vi "Polynomial Roots (CDB).vi"(10 "option":u16(ring) items=["General"=0, "Advanced Refinement"=3], 11 "P(x)":cdb[](array[numeric]) format="%#.6g") -> (0 "error":i32, 3 "Roots":cdb[](array[numeric]) format="%#.6g")   [LabVIEW 2010, in "NI_AALPro.lvlib"]
doc: "Finds the roots of polynomial <B>P(x)</B>. This VI removes leading coefficients of the polynomial that are equal to zero. Wire data to the <B>P(x)</B> input to determine the polymorphic instance to use or manually select the instance."
uses:
  NI_AALPro.lvlib
  Remove Zero Coefficients (CDB).vi
  lvanlys.dll
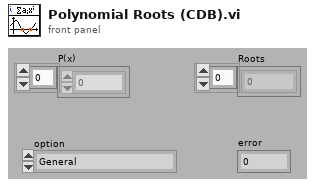
[diagram p1: front panel]
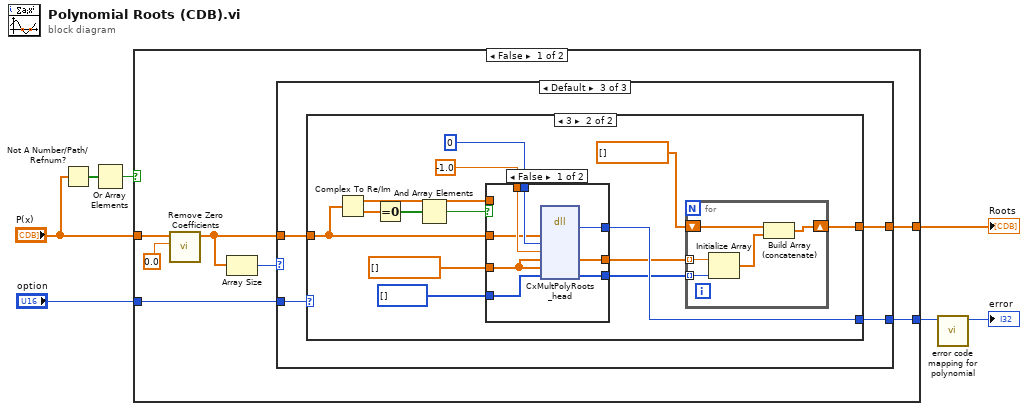
[diagram p0: block diagram]
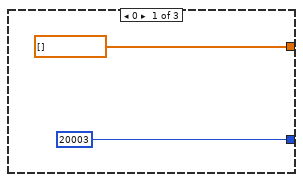
[diagram p2: hidden frame]
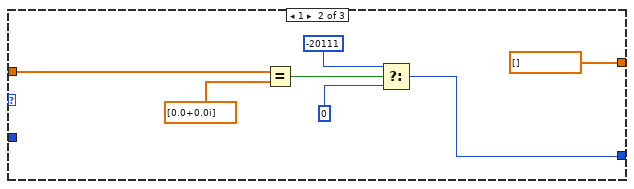
[diagram p3: hidden frame]
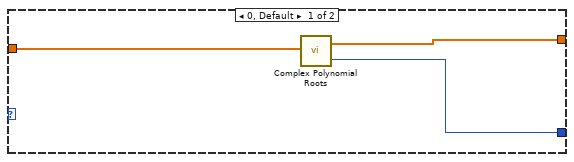
[diagram p4: hidden frame]
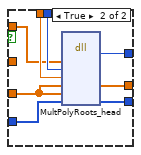
[diagram p5: hidden frame]
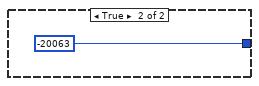
[diagram p6: hidden frame]
diagram:
  n1 = Not A Number/Path/Refnum?(number/path/refnum="P(x)") -> (NaN/Path/Refnum?=w1:bool[])
  n2 = Or Array Elements(Boolean array=w1) -> (logical OR=w2:bool)
  n3 = case shown="False" w2 {
    tunnel: [w14 _] -> w7
    tunnel: "option" -> [w12 _]
    tunnel: [w11 -20063 ("error")] -> w5
    tunnel: "P(x)" -> [w9 _]
    frame False {
      n4 = call-poly "Remove Zero Coefficients.vi"("threshold"=0.0, "P(x) In"=w9) -> ("P(x) Out"=w8:cdb[])  [unwired: 1 in, 8 out]
      n5 = Array Size(array=w8) -> (size(s)=w13:i32)
      n6 = case shown="Default" w13 {
        tunnel: [cdb[] [] ("Polynomial Roots") cdb[] [] ("Approximate Roots") w27] -> w14
        tunnel: [20003 ("empty array") w17 w25] -> w11
        tunnel: w8 -> [_ w22 w24]
        tunnel: w12 -> [_ _ w26]
        frame 0 {
        }
        frame 1 {
          n7 = Equal?(x=w22, y=cdb[] [0.0+0.0i]) -> (x = y?=w20:bool)
          n8 = Select(t=-20111, s=w20, f=0) -> (s? t:f=w17:i32)
        }
        frame Default {
          n9 = case shown="3" w26 {
            tunnel: [w29 w43] -> w27
            tunnel: w24 -> [w30 w35]
            tunnel: [w28 w42] -> w25
            frame 0, Default {
              n10 = call "Complex Polynomial Roots.vi"("Polynomial"=w30) -> ("Polynomial Roots"=w29:cdb[], "error"=w28:i32)
            }
            frame 3 {
              n11 = Complex To Re/Im(x + iy=w35) -> (x=w31:dbl[], y=w34:dbl[])
              n12 = Equal To 0?(x=w34) -> (x = 0?=w33:bool[])
              n13 = And Array Elements(Boolean array=w33) -> (logical AND=w32:bool)
              n14 = case shown="False" w32 {
                tunnel: [w52 w55] -> w42
                tunnel: i32[] [] -> [w51 w56]
                tunnel: [w50 w53] -> w40
                tunnel: cdb[] [] ("Roots") -> [w49 w57]
                tunnel: [w48 w54] -> w38
                tunnel: -1.0 ("tol") -> [w47 w59]
                tunnel: 0 ("alg2") -> [w46 w60]
                tunnel: w35 -> [w45 _]
                tunnel: w31 -> [_ w58]
                frame False {
                  n15 = dll-call lib="C:/Program Files/National Instruments/LabVIEW 2010/resource/lvanlys.*" fn="CxMultPolyRoots_head"("pH"=w45, "alg2"=w46, "tol"=w47, "approotH"=w49, "rootH"=w49, "multH"=w51) -> ("return type"=w52:i32, "approotH"=w48:cdb[], "multH"=w50:i32[])  [unwired: 7 in, 2 out]
                }
                frame True {
                  n16 = dll-call lib="C:/Program Files/National Instruments/LabVIEW 2010/resource/lvanlys.*" fn="MultPolyRoots_head"("pH"=w58, "alg2"=w60, "tol"=w59, "appRootH"=w57, "rootH"=w57, "multH"=w56) -> ("return type"=w55:i32, "appRootH"=w54:cdb[], "multH"=w53:i32[])  [unwired: 7 in, 2 out]
                }
              }
              n17 = for {
                shift-right: [w61] -> w43
                shift-left: cdb[] [] ("Approximate Roots") -> [w62]
                tunnel: w40 -> [w65] mode=indexing
                tunnel: w38 -> [w64] mode=indexing
                n18 = Initialize Array(w64, w65) -> (w63:cdb[])
                n19 = Build Array (concatenate)(w62, w63) -> (w61:cdb[])
              }
            }
          }
        }
      }
    }
    frame True {
    }
  }
  "Roots" <- w7
  n20 = call "error code mapping for polynomial.vi"("error in"=w5) -> ("error out"=→"error":i32)  [unwired: 10 out]
